vi "Intake_Set.vi"   [LabVIEW 2019]
uses:
  Globals/Intake_Globals.vi
types:
  T1 = typedef "Intake_Cluster.ctl" = cluster{"Control_State":enum16{"Manual_Control"}, "Intake_On":bool, "Intake_Extended":bool}
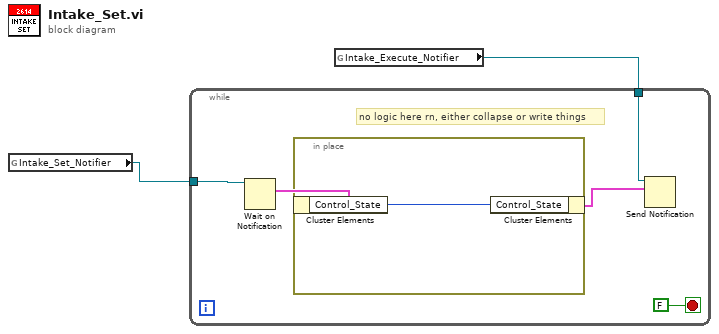
[diagram p0: block diagram]
diagram:
  n1 = global read "Intake_Globals.vi" "Intake_Set_Notifier"() -> (w2:refnum<notifier>)
  n2 = global read "Intake_Globals.vi" "Intake_Execute_Notifier"() -> (w1:refnum<notifier>)
  n3 = while {
    tunnel: w2 -> [w6]
    tunnel: w1 -> [w4]
    stop <- FALSE stop-if-true
    # "no logic here rn, either collapse or write things"
    n4 = Wait on Notification(notifier=w6) -> (notification=w5:T1)  [unwired: 3 in, 3 out]
    n5 = in-place {
      n6 = in-place-cluster #1(w5) -> ("Control_State"=w8:enum16{"Manual_Control"})
      n7 = in-place-cluster #1("Control_State"=w8) -> (w3:T1)
    }
    n8 = Send Notification(notification=w3, notifier=w4) -> ()  [unwired: 1 in, 2 out]
  }
